vi "HRTF-Read Response.vi"(2 "State":T1, 7 "filestem":string, 11 "error in (no error)":errorcluster) -> (6 "time":cluster{"offset":dbl, "dx":dbl, "Y":dbl[][]}, 8 "crosscorr":cluster{"offset":dbl, "dx":dbl, "Y":dbl[][]}, 13 "phase":cluster{"offset":dbl, "dx":dbl, "Y":dbl[][]}, 14 "mag":cluster{"offset":dbl, "dx":dbl, "Y":dbl[][]}, 15 "error out":errorcluster)   [LabVIEW 2015]
uses:
  Typedefs/HRTF-State.ctl
  Typedefs/HRTF-Laterality.ctl
  Typedefs/HRTF-Parameters.ctl
  Typedefs/HRTF-Waveform.ctl
  <vilib>/Analysis/2dsp.llb/Complex FFT.vi
  <vilib>/Analysis/2dsp.llb/Inverse Real FFT.vi
  Utility VIs/Math VIs/FFT x(t) to dB,Degrees (1D).vi
  Utility VIs/Conversion VIs/Create Waveform Cluster (2D).vi
  PXI DAQ VIs/Utility VIs/Array Dimensions (2D).vi
  <vilib>/Analysis/NI_AALPro.lvlib
panel:
  out "error out":errorcluster
  in  "Result":cluster{"Stimulus":dbl[], "Response":dbl[]}
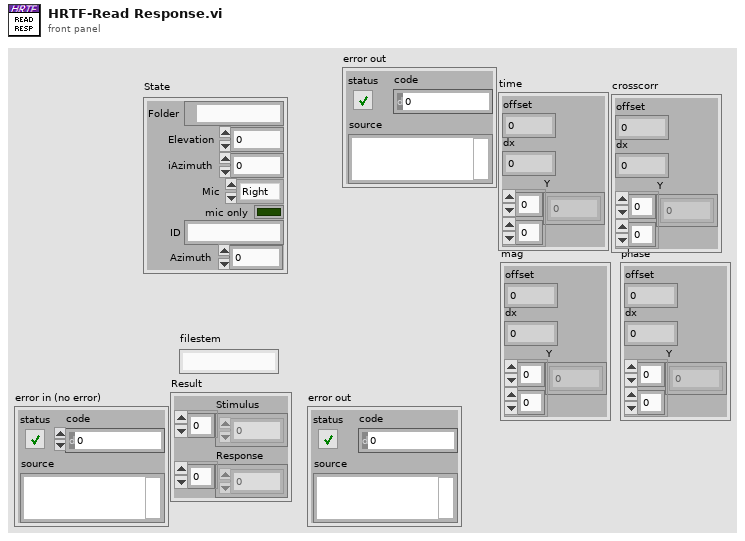
[diagram p1: front panel]
types:
  T1 = typedef "HRTF-State.ctl" = cluster{"Folder":path, "Elevation":dbl, "iAzimuth":i32, "Mic":T2, "mic only":bool, "ID":string, "Azimuth":dbl}
  T2 = typedef "HRTF-Laterality.ctl" = enum16{"Right", "Left"}
  T3 = typedef "HRTF-Parameters.ctl" = cluster{"Fs (Hz)":dbl, "atten (dB)":dbl, "Waveform":T4, "Freq Res (Hz)":dbl, "Order":i32, "Gain (dB)":dbl, "Averages":i32, "seed":i64}
  T4 = typedef "HRTF-Waveform.ctl" = enum16{"Chirp", "MLS"}
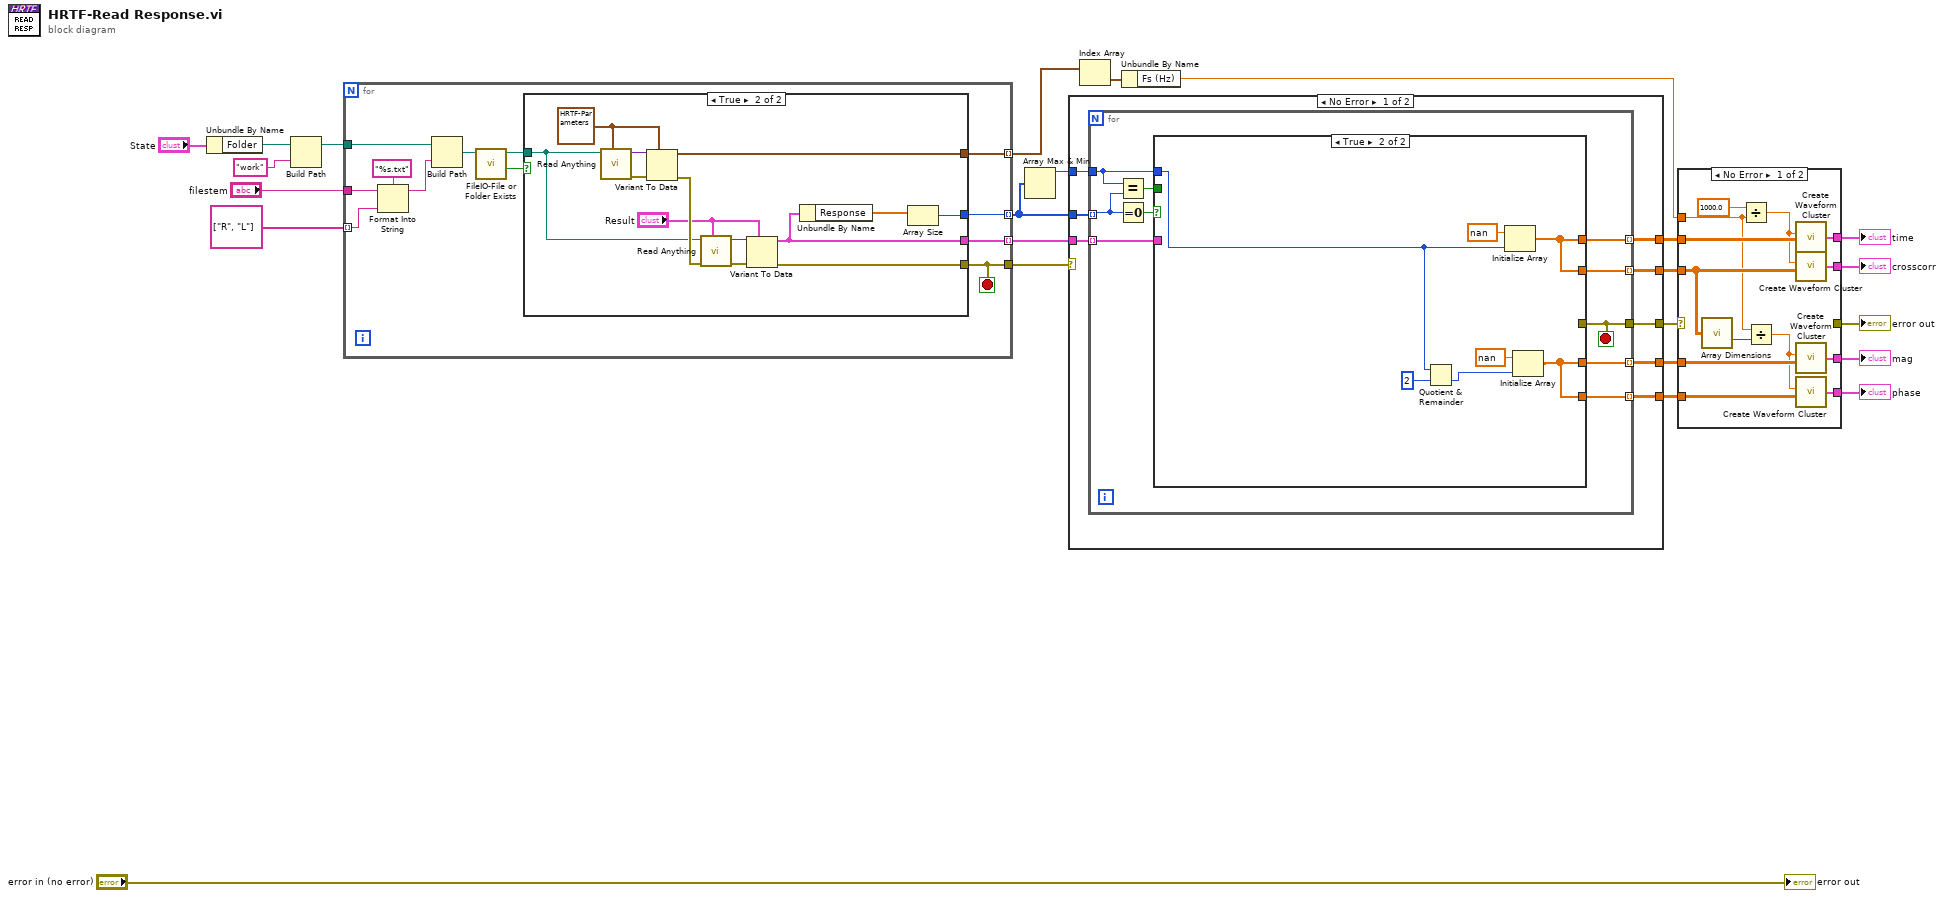
[diagram p0: block diagram]
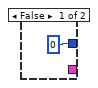
[diagram p3: hidden frame]
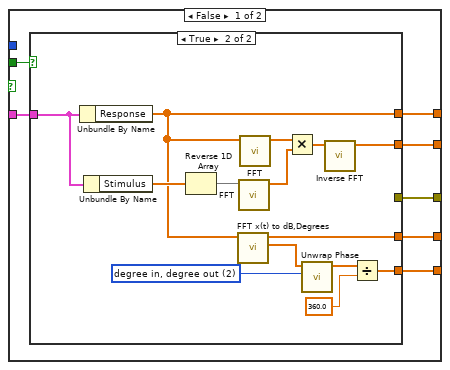
[diagram p4: hidden frame]
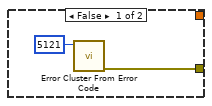
[diagram p5: hidden frame]
diagram:
  n1 = Unbundle By Name("State") -> ("Folder"=w21:path)
  n2 = Build Path(base path=w21, name or relative path="work") -> (appended path=w2:path)
  n3 = for {
    tunnel: string[] ["R", "L"] -> [w34] mode=indexing
    tunnel: w2 -> [w33]
    tunnel: "filestem" -> [w36]
    tunnel: [w31] -> w5 mode=indexing
    tunnel: [w30] -> w18 mode=indexing
    tunnel: [w25] -> w19
    tunnel: [w26] -> w16 mode=indexing
    stop <- w25 stop-if-true
    n4 = Format Into String(format string="%s.txt", initial string=w36, w34) -> (resulting string=w32:string)  [unwired: 1 in, 1 out]
    n5 = Build Path(base path=w33, name or relative path=w32) -> (appended path=w29:path)
    n6 = call "FileIO-File or Folder Exists.vi"("path"=w29) -> ("Exists?"=w27:bool, "dup path"=w28:path)  [unwired: 7 in, 2 out]
    n7 = case shown="True" w27 {
      tunnel: [_ w41] -> w31
      tunnel: w28 -> [_ w43]
      tunnel: [_ w39] -> w30
      tunnel: [_ w42] -> w25
      tunnel: [0 w40] -> w26
      frame False {
      }
      frame True {
        w48 = T3 {"Fs (Hz)"=0.0, "atten (dB)"=0.0, "Waveform"=enum."Chirp", "Freq Res (Hz)"=0.0, "Order"=0, "Gain (dB)"=0.0, "Averages"=0, "seed"=-1} ("Params")
        n8 = call "Read Anything.vi"("Type of Anything"=w48, "Path (dialog)"=w43) -> ("Error Out"=w50:errorcluster, "Anything"=w49:variant)  [unwired: 7 in, 1 out]
        n9 = Variant To Data(error in=w50, type=w48, Variant=w49) -> (data=w41:T3, error out=w46:errorcluster)
        n10 = call "Read Anything.vi"("Type of Anything"="Result", "Error In"=w46, "Path (dialog)"=w43) -> ("Error Out"=w47:errorcluster, "Anything"=w44:variant)  [unwired: 6 in, 1 out]
        n11 = Variant To Data(error in=w47, type="Result", Variant=w44) -> (data=w39:cluster{"Stimulus":dbl[], "Response":dbl[]}, error out=w42:errorcluster)
        n12 = Unbundle By Name(w39) -> ("Response"=w38:dbl[])
        n13 = Array Size(array=w38) -> (size(s)=w40:i32)
      }
    }
  }
  n14 = Array Max & Min(array=w16) -> (max value=w17:i32)  [unwired: 3 out]
  n15 = case shown="No Error" w19 {
    selector: w19 -> [_ w99]
    tunnel: w18 -> [w58 _]
    tunnel: w17 -> [w57 _]
    tunnel: w16 -> [w56 _]
    tunnel: [w55 w99] -> w15
    tunnel: [w54 _] -> w13
    tunnel: [w53 _] -> w14
    tunnel: [w52 _] -> w12
    tunnel: [w51 _] -> w11
    frame No Error {
      n16 = for {
        tunnel: w58 -> [w64] mode=indexing
        tunnel: w57 -> [w67]
        tunnel: w56 -> [w66] mode=indexing
        tunnel: [w63] -> w54 mode=indexing
        tunnel: [w62] -> w53 mode=indexing
        tunnel: [w61] -> w52 mode=indexing
        tunnel: [w60] -> w51 mode=indexing
        tunnel: [w59] -> w55
        stop <- w59 stop-if-true
        n17 = Equal?(x=w67, y=w66) -> (x = y?=w65:bool)
        n18 = Equal To 0?(x=w66) -> (x = 0?=w68:bool)
        n19 = case shown="True" w68 {
          tunnel: w67 -> [_ w94]
          tunnel: w65 -> [w75 _]
          tunnel: w64 -> [w74 _]
          tunnel: [w73 w97] -> w63
          tunnel: [w72 w97] -> w62
          tunnel: [w71 w95] -> w61
          tunnel: [w70 w95] -> w60
          tunnel: [w69 _] -> w59
          frame False {
            n20 = case shown="True" w75 {
              tunnel: w74 -> [_ w83]
              tunnel: [_ w81] -> w73
              tunnel: [_ w80] -> w72
              tunnel: [_ w79] -> w71
              tunnel: [_ w78] -> w70
              tunnel: [w76 _] -> w69
              frame False {
                n21 = call <vilib>:"Error Cluster From Error Code.vi"("error code (0)"=5121) -> ("error out"=w76:errorcluster)  [unwired: 8 in]
              }
              frame True {
                w89 = 2 items=["radian in, radian out", "radian in, degree out", "degree in, degree out", "degree in, radian out"] ("phase unit")
                n22 = Unbundle By Name(w83) -> ("Response"=w81:dbl[])
                n23 = Unbundle By Name(w83) -> ("Stimulus"=w86:dbl[])
                n24 = Reverse 1D Array(array=w86) -> (reversed array=w87:dbl[])
                n25 = call-poly "FFT x(t) to dB,Degrees.vi"("X"=w81) -> ("+Freq Phase of FFT (degrees)"=w90:dbl[], "+Freq. Mag of FFT (dB rms)"=w79:dbl[])  [unwired: 8 in, 1 out]
                n26 = call-poly <vilib>:"FFT.vi"("X"=w87) -> ("FFT {X}"=w88:cdb[])  [unwired: 9 in, 1 out]
                n27 = call-poly <vilib>:"FFT.vi"("X"=w81) -> ("FFT {X}"=w85:cdb[])  [unwired: 9 in, 1 out]
                n28 = Multiply(x=w85, y=w88) -> (x*y=w84:cdb[])
                n29 = call <vilib>:"Unwrap Phase.vi"("phase unit"=w89, "Phase"=w90) -> ("Unwrapped Phase"=w91:dbl[])  [unwired: 8 in, 1 out]
                n30 = call-poly <vilib>:"Inverse FFT.vi"("FFT {X}"=w84) -> ("X"=w80:dbl[])  [unwired: 9 in, 1 out]
                n31 = Divide(x=w91, y=360.0) -> (x/y=w78:dbl[])
              }
            }
          }
          frame True {
            n32 = Quotient & Remainder(x=w94, y=2) -> (floor(x/y)=w92:i32)  [unwired: 1 out]
            n33 = Initialize Array(nan, w94) -> (w97:dbl[])
            n34 = Initialize Array(nan, w92) -> (w95:dbl[])
          }
        }
      }
    }
    frame Error {
    }
  }
  n35 = Index Array(array=w5) -> (element=w4:T3)  [unwired: 1 in]
  n36 = Unbundle By Name(w4) -> ("Fs (Hz)"=w3:dbl)
  n37 = case shown="No Error" w15 {
    selector: w15 -> [_ w113]
    tunnel: w14 -> [w103 _]
    tunnel: w13 -> [w112 _]
    tunnel: w12 -> [w111 _]
    tunnel: w11 -> [w110 _]
    tunnel: [w109 _] -> w10
    tunnel: [w108 _] -> w9
    tunnel: [w107 _] -> w8
    tunnel: [w106 _] -> w7
    tunnel: [_ w113] -> w6
    tunnel: w3 -> [w101 _]
    frame No Error {
      n38 = call-poly "Array Dimensions.vi"("2D Array"=w103) -> ("# columns"=w102:i32)  [unwired: 13 in, 1 out]
      n39 = Divide(x=1000.0, y=w101) -> (x/y=w104:dbl)
      n40 = Divide(x=w101, y=w102) -> (x/y=w100:dbl)
      n41 = call-poly "Create Waveform Cluster.vi"("dx"=w104, "Array"=w112) -> ("waveform cluster"=w109:cluster{"offset":dbl, "dx":dbl, "Y":dbl[][]})  [unwired: 3 in]
      n42 = call-poly "Create Waveform Cluster.vi"("dx"=w104, "Array"=w103) -> ("waveform cluster"=w108:cluster{"offset":dbl, "dx":dbl, "Y":dbl[][]})  [unwired: 3 in]
      n43 = call-poly "Create Waveform Cluster.vi"("dx"=w100, "Array"=w111) -> ("waveform cluster"=w107:cluster{"offset":dbl, "dx":dbl, "Y":dbl[][]})  [unwired: 3 in]
      n44 = call-poly "Create Waveform Cluster.vi"("dx"=w100, "Array"=w110) -> ("waveform cluster"=w106:cluster{"offset":dbl, "dx":dbl, "Y":dbl[][]})  [unwired: 3 in]
    }
    frame Error {
    }
  }
  "time" <- w10
  "mag" <- w8
  "phase" <- w7
  "crosscorr" <- w9
  "error out" <- w6
  "error out" <- "error in (no error)"
